vi "Get MetaData from Results.vi"(8 "error in":errorcluster, 11 "Configuration Cluster":variant) -> (0 "error out":errorcluster, 3 "outputs":T1[](array[typedef]))   [LabVIEW 2020, in "Line Regulation.lvlib"]
uses:
  Line Regulation.lvlib
  RPC Messages/ni_measurements_v1_Output.ctl
  <vilib>/Utility/Data Type/NI_Data Type.lvlib
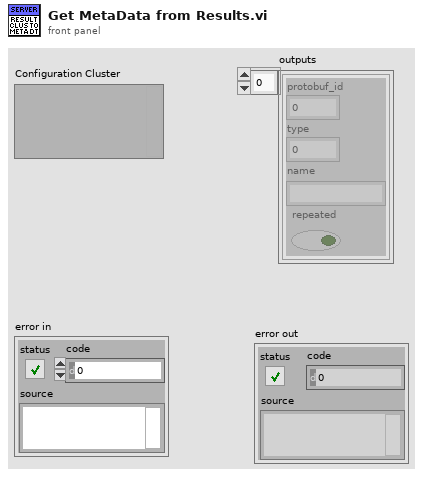
[diagram p1: front panel]
types:
  T1 = typedef "Line Regulation.lvlib/ni_measurements_v1_Output.ctl" = cluster{"protobuf_id":u32, "type":i32, "name":string, "repeated":bool}
  T2 = typedef "NI_Data Type.lvlib/Data Type.ctl" = enum8{"Invalid Type", "Void", "I8", "I16", "I32", "I64", "U8", "U16", "U32", "U64", "Single Float", "Double Float", "Extended Float", "Single Complex", "Double Complex", "Extended Complex", "Enum U8", "Enum U16", "Enum U32", "Enum U64", "Single Float With Unit", "Double Float With Unit", "Extended Float With Unit", "Single Complex with Unit", "Double Complex with Unit", "Extended Complex with Unit", "Boolean", "String", "Path", "Picture", "Tag", "Array", "Cluster", "Variant", "LV Variant", "Waveform", "Timestamp", "Digital Waveform", "Digital Data", "ExpressData", "Refnum", "External Data", "VI", "Poly VI", "LabVIEW Class Instance", "Fixed Point", "Set Collection", "Map Collection"}
  T3 = typedef "Line Regulation.lvlib/ni_measurements_v1_Type.ctl" = enum32{"TYPE_UNSPECIFIED", "TYPE_DOUBLE", "TYPE_FLOAT", "TYPE_INT64", "TYPE_UINT64", "TYPE_INT32", "TYPE_FIXED64", "TYPE_FIXED32", "TYPE_BOOL", "TYPE_STRING", "TYPE_GROUP", "TYPE_MESSAGE", "TYPE_BYTES", "TYPE_UINT32", "TYPE_ENUM", "TYPE_SFIXED32", "TYPE_SFIXED64", "TYPE_SINT32", "TYPE_SINT64"}
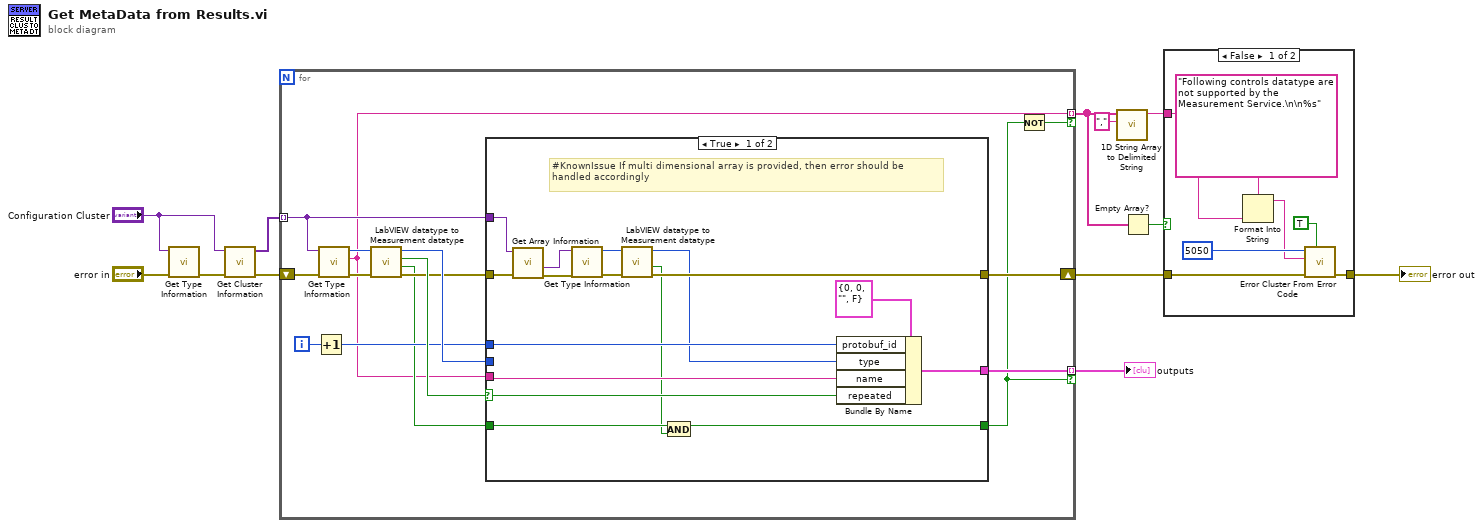
[diagram p0: block diagram]
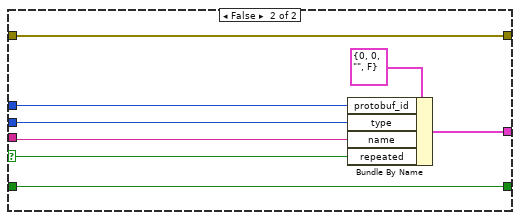
[diagram p3: hidden frame]
diagram:
  n1 = call <vilib>:"Get Type Information.vi"("error in (no error)"="error in", "variant"="Configuration Cluster") -> ("error out"=w12:errorcluster)  [unwired: 5 in, 4 out]
  n2 = call <vilib>:"Get Cluster Information.vi"("error in (no error)"=w12, "variant"="Configuration Cluster") -> ("error out"=w10:errorcluster, "cluster elements"=w11:variant[])  [unwired: 8 in]
  n3 = for {
    tunnel: w11 -> [w21] mode=indexing
    tunnel: [w22] -> w9 mode=indexing if=w14
    shift-right: [w17] -> w7
    shift-left: w10 -> [w27]
    tunnel: [w15] -> w6 mode=indexing if=w13
    i -> [w26]
    n4 = Increment(x=w26) -> (x+1=w18:i32)
    n5 = call <vilib>:"Get Type Information.vi"("error in (no error)"=w27, "variant"=w21) -> ("error out"=w20:errorcluster, "name"=w15:string, "type"=w25:T2)  [unwired: 5 in, 2 out]
    n6 = call "LabVIEW datatype to Measurement datatype.vi"("error in"=w20, "type"=w25) -> ("error out"=w19:errorcluster, "Supported?"=w16:bool, "Array?"=w23:bool, "MessageElementType"=w24:T3)  [unwired: 6 in]
    n7 = case shown="True" w23 {
      selector: w23 -> [w43 w51]
      tunnel: w18 -> [w34 w48]
      tunnel: w24 -> [_ w46]
      tunnel: [w42 w50] -> w22
      tunnel: w19 -> [w41 w49]
      tunnel: w21 -> [w40 _]
      tunnel: [w36 w49] -> w17
      tunnel: w15 -> [w32 w47]
      tunnel: w16 -> [w30 w44]
      tunnel: [w29 w44] -> w14
      frame True {
        # "#KnownIssue If multi dimensional array is provided, then error should be handled accordingly"
        n8 = call <vilib>:"Get Array Information.vi"("error in (no error)"=w41, "variant"=w40) -> ("error out"=w39:errorcluster, "array element data type"=w35:variant)  [unwired: 6 in, 2 out]
        n9 = call <vilib>:"Get Type Information.vi"("error in (no error)"=w39, "variant"=w35) -> ("error out"=w37:errorcluster, "type"=w38:T2)  [unwired: 5 in, 3 out]
        n10 = call "LabVIEW datatype to Measurement datatype.vi"("error in"=w37, "type"=w38) -> ("error out"=w36:errorcluster, "Supported?"=w28:bool, "MessageElementType"=w33:T3)  [unwired: 6 in, 1 out]
        n11 = And(x=w30, y=w28) -> (x .and. y?=w29:bool)
        n12 = Bundle By Name(cluster=T1 {"protobuf_id"=0, "type"=0, "name"="", "repeated"=FALSE} ("ni_measurements_v1_Output"), "protobuf_id"=w34, "type"=w33, "name"=w32, "repeated"=w43) -> (w42:T1)
      }
      frame False {
        n13 = Bundle By Name(cluster=T1 {"protobuf_id"=0, "type"=0, "name"="", "repeated"=FALSE} ("ni_measurements_v1_Output"), "protobuf_id"=w48, "type"=w46, "name"=w47, "repeated"=w51) -> (w50:T1)
      }
    }
    n14 = Not(x=w14) -> (.not. x?=w13:bool)
  }
  "outputs" <- w9
  n15 = call <vilib>:"1D String Array to Delimited String.vi"("delimiter"=",", "string array"=w6) -> ("delimited string"=w4:string)  [unwired: 9 in]
  n16 = Empty Array?(array=w6) -> (empty?=w5:bool)
  n17 = case shown="False" w5 {
    tunnel: w7 -> [w58 w59]
    tunnel: [w57 w59] -> w1
    tunnel: w4 -> [w54 _]
    frame False {
      n18 = Format Into String(format string="Following controls datatype are not supported by the Measurement Service.\n\n%s", w54) -> (resulting string=w53:string)  [unwired: 2 in, 1 out]
      n19 = call <vilib>:"Error Cluster From Error Code.vi"("show call chain? (False)"=TRUE, "error in (no error)"=w58, "error message (\"\")"=w53, "error code (0)"=5050) -> ("error out"=w57:errorcluster)  [unwired: 5 in]
    }
    frame True {
    }
  }
  "error out" <- w1
